vi "readFromXML.vi"(8 "error in (no error)":errorcluster, 10 "XML in":string, 11 "MccDisable in":refnum<class "MccDisable.lvclass">) -> (0 "error out":errorcluster, 3 "MccDisable out":refnum<class "MccDisable.lvclass">)   [LabVIEW 2022 SP3, in "TCSDataDefinitions.lvlib" / "TCSMountControlCommand.lvlib" / "CommandsForAllAxes.lvlib" / "MccDisable.lvclass"]
uses:
  MccDisable.lvclass
  CommandsForAllAxes.lvclass
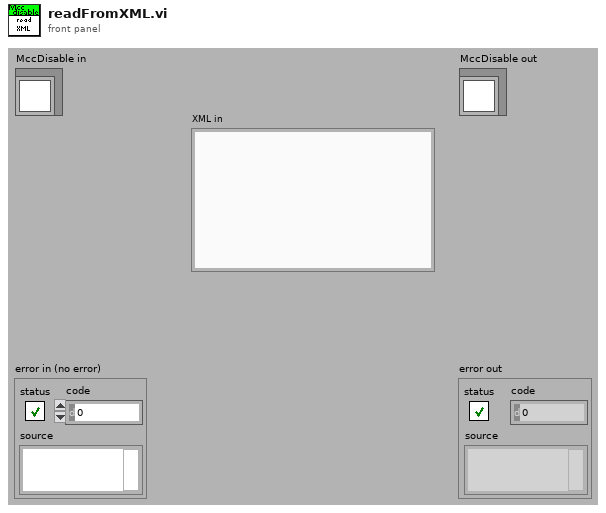
[diagram p1: front panel]
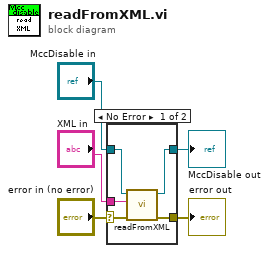
[diagram p0: block diagram]
diagram:
  n1 = case shown="No Error" "error in (no error)" {
    selector: "error in (no error)" -> [w8 w12]
    tunnel: [w7 w12] -> w4
    tunnel: [w9 w11] -> w2
    tunnel: "MccDisable in" -> [w10 w11]
    tunnel: "XML in" -> [w6 _]
    frame No Error {
      n2 = call-parent "readFromXML.vi"("error in (no error)"=w8, "XML in"=w6, "CommandsForAllAxes in"=w10) -> ("error out"=w7:errorcluster, "CommandsForAllAxes out"=w9:refnum<class "MccDisable.lvclass">)  [unwired: 7 out]
    }
    frame Error {
    }
  }
  "error out" <- w4
  "MccDisable out" <- w2
